vi "Affichage_Graphiques.vi"(10 "Poids":i32, 11 "Position":i32) -> (1 "Graphique 2 Poids en fonction du temps":dbl[](array[numeric]), 2 "Etage Actuel":dbl, 3 "Graphique 1 Position en fonction du temps":dbl[](array[numeric]), 4 "Poids cabine":dbl)   [LabVIEW 2026]
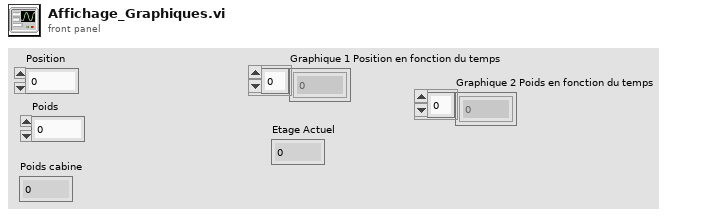
[diagram p1: front panel]
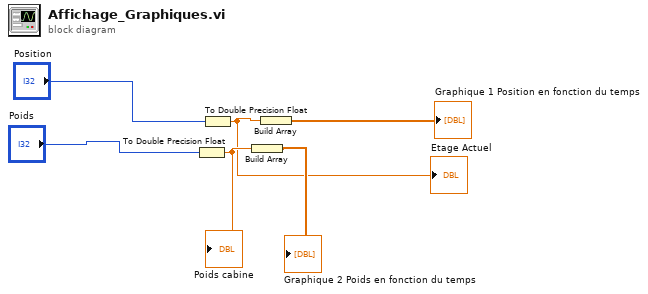
[diagram p0: block diagram]
diagram:
  n1 = To Double Precision Float(number="Poids") -> (double precision float=w3:dbl)
  "Poids cabine" <- w3
  n2 = To Double Precision Float(number="Position") -> (double precision float=w2:dbl)
  "Etage Actuel" <- w2
  n3 = Build Array(w3) -> (→"Graphique 2 Poids en fonction du temps":dbl[])
  n4 = Build Array(w2) -> (→"Graphique 1 Position en fonction du temps":dbl[])
